vi "Set Log File Specification Path Tag.vi"(8 "error in (no error)":errorcluster, 9 "Value":string, 10 "Path Tag":string, 11 "Segmented Log in":refnum<class "Segmented Log.lvclass">) -> (0 "error out":errorcluster, 3 "Segmented Log out":refnum<class "Segmented Log.lvclass">)   [LabVIEW 2015, in "Segmented Log.lvclass"]
doc: "Sets a path tag on the contained Log File Specification instance."
uses:
  Segmented Log.lvclass
  Segmented Log.lvclass/Segmented Log.ctl
  Log File Specifications/Log File Specification/Log File Specification.lvclass/Log File Specification.ctl
  Log File Specifications/Log File Specification/Log File Specification.lvclass
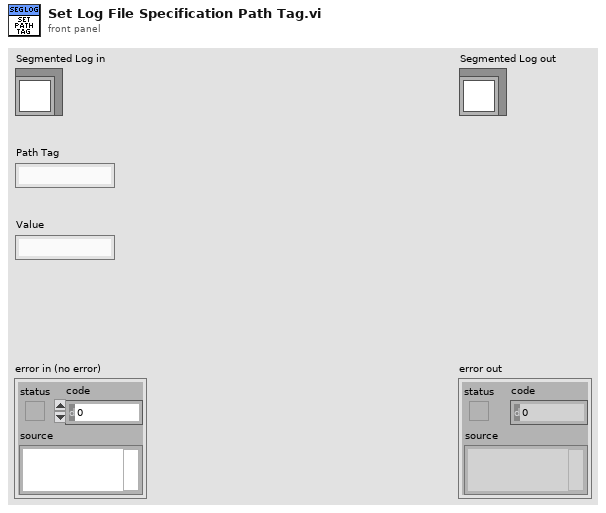
[diagram p1: front panel]
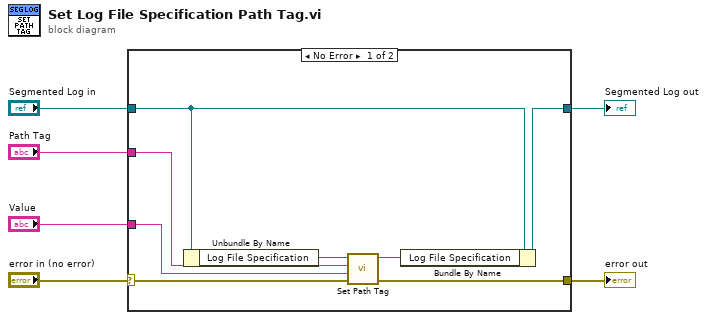
[diagram p0: block diagram]
diagram:
  n1 = case shown="No Error" "error in (no error)" {
    selector: "error in (no error)" -> [w7 w15]
    tunnel: "Segmented Log in" -> [w14 w16]
    tunnel: [w12 w16] -> w5
    tunnel: [w10 w15] -> w4
    tunnel: "Path Tag" -> [w9 _]
    tunnel: "Value" -> [w8 _]
    frame No Error {
      n2 = Unbundle By Name(w14) -> ("Log File Specification"=w13:refnum<class "Log File Specification.lvclass">)
      n3 = call "Set Path Tag.vi"("error in (no error)"=w7, "Tag Value"=w8, "Tag Name"=w9, "Log File Specification in"=w13) -> ("error out"=w10:errorcluster, "Log File Specification out"=w11:refnum<class "Log File Specification.lvclass">)  [unwired: 6 in]
      n4 = Bundle By Name(cluster=w14, "Log File Specification"=w11) -> (w12:refnum<class "Segmented Log.lvclass">)
    }
    frame Error {
    }
  }
  "error out" <- w4
  "Segmented Log out" <- w5
